vi "generate.vi"(0 "lower bound":u32, 7 "upper bound":u32=100, 11 "Error in":errorcluster) -> (6 "Generated number":u32, 15 "Error out":errorcluster)   [LabVIEW 2020]
doc: "This VI is used to generate random number from random number genrator within the range"
panel:
  # "GENERATE DATA"
  # "INPUT"
  # "OUTPUT"
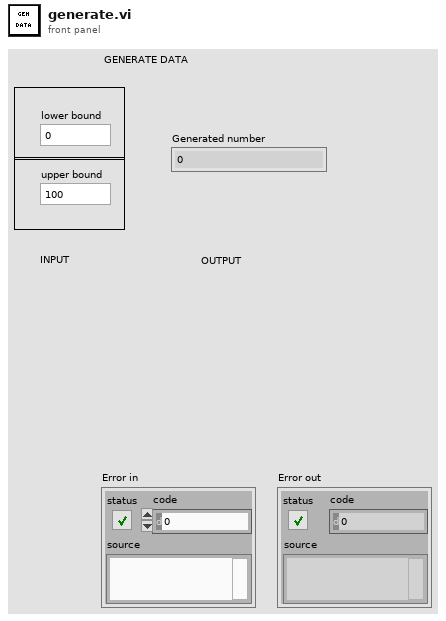
[diagram p1: front panel]
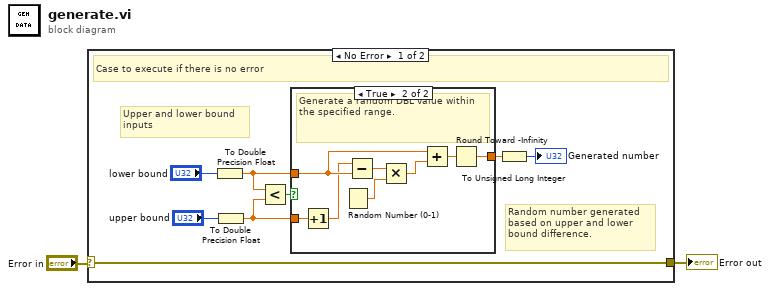
[diagram p0: block diagram]
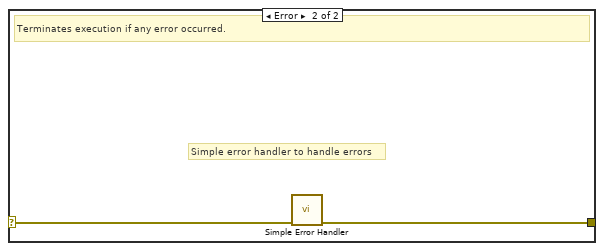
[diagram p3: hidden frame]
diagram:
  n1 = case shown="No Error" "Error in" {
    selector: "Error in" -> [w3 w21]
    tunnel: [w3 w20] -> w1
    frame No Error {
      # "Upper and lower bound\ninputs"
      # "Random number generated\nbased on upper and lower \nbound difference."
      # "Case to execute if there is no error"
      n2 = To Double Precision Float(number="lower bound") -> (double precision float=w8:dbl)
      n3 = To Double Precision Float(number="upper bound") -> (double precision float=w9:dbl)
      n4 = Less?(x=w8, y=w9) -> (x < y?=w4:bool)
      n5 = case shown="True" w4 {
        tunnel: w8 -> [w11 w16]
        tunnel: w9 -> [_ w19]
        tunnel: [w11 w12] -> w7
        frame False {
          # "If bounds are reversed, always return the lower bound."
        }
        frame True {
          # "Generate a random DBL value within the specified range."
          n6 = Increment(x=w19) -> (x+1=w13:dbl)
          n7 = Random Number (0-1)() -> (number: 0 to 1=w17:dbl)
          n8 = Subtract(x=w13, y=w16) -> (x-y=w18:dbl)
          n9 = Multiply(x=w18, y=w17) -> (x*y=w15:dbl)
          n10 = Add(x=w16, y=w15) -> (x+y=w14:dbl)
          n11 = Round Toward -Infinity(1:w14) -> (0:w12:dbl)
        }
      }
      n12 = To Unsigned Long Integer(number=w7) -> (unsigned 32bit integer=→"Generated number":u32)
    }
    frame Error {
      # "Simple error handler to handle errors"
      # "Terminates execution if any error occurred."
      n13 = call <vilib>:"Simple Error Handler.vi"("error in (no error)"=w21) -> ("error out"=w20:errorcluster)  [unwired: 4 in, 4 out]
    }
  }
  "Error out" <- w1
